vi "Clear Framebuffer.vi"(11 "Pixel Data in":u32[][](array[numeric])) -> (3 "Pixel Data out":u32[][](array[numeric]))   [LabVIEW 2022 SP3, in "Raster.lvlib"]
uses:
  Raster.lvlib
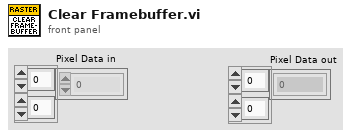
[diagram p1: front panel]
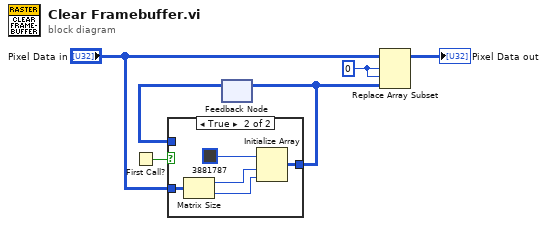
[diagram p0: block diagram]
diagram:
  w4 = 0 ("index (row)")
  n1 = First Call?() -> (First Call?: T/F=w3:bool)
  n2 = feedback #1() -> (w1:u32[][])  [unwired: 1 in]
  n3 = case shown="True" w3 {
    tunnel: "Pixel Data in" -> [_ w12]
    tunnel: [w7 w11] -> w2
    tunnel: w1 -> [w7 _]
    frame False {
    }
    frame True {
      n4 = Matrix Size(0:w12) -> (1:w10:i32, 2:w9:i32)
      n5 = Initialize Array(u32 3881787 ("Fill Colour"), w10, w9) -> (w11:u32[][])
    }
  }
  n6 = feedback-in #1(w2) -> ()
  n7 = Replace Array Subset(array="Pixel Data in", new element=w2, index (row)=w4, index (col)=w4) -> (→"Pixel Data out":u32[][])
